vi "FPGA_Amplitude_Pockels_Galvo.vi"(5 "Live(F)/Functional(T)":bool, 6 "Chirp index":i32, 7 "FPGA Type":enum16{"Virtex 5", "Virtex 7"}(ring), 8 "delta_a_dz":dbl[](array[numeric]), 9 "difftime - aodcontrol delay":dbl, 10 "Laser(V) - Vertex 7 Only":dbl[](array[numeric]), 11 "Amplitude":dbl[](array[numeric])) -> (2 "Pockels_Galvo_Params":T1)   [LabVIEW 2020]
uses:
  Controls/Pockels_Galvo_Params.ctl
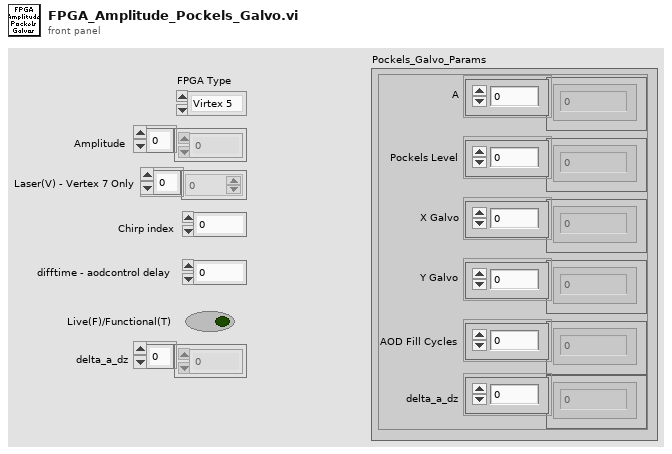
[diagram p1: front panel]
types:
  T1 = typedef "Pockels_Galvo_Params.ctl" = cluster{"A":dbl[], "Pockels Level":dbl[], "X Galvo":dbl[], "Y Galvo":dbl[], "AOD Fill Cycles":dbl[], "delta_a_dz":dbl[]}
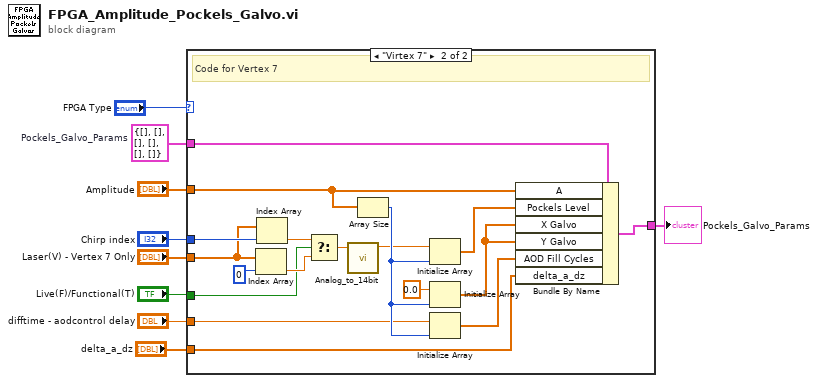
[diagram p0: block diagram]
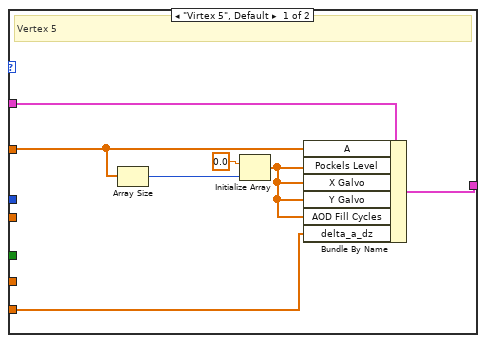
[diagram p2: hidden frame]
diagram:
  w9 = T1 {"A"=[], "Pockels Level"=[], "X Galvo"=[], "Y Galvo"=[], "AOD Fill Cycles"=[], "delta_a_dz"=[]}  # Pockels_Galvo_Params
  n1 = case shown="\"Virtex 7\"" "FPGA Type" {
    tunnel: w9 -> [w15 w25]
    tunnel: "Amplitude" -> [w12 w24]
    tunnel: "Chirp index" -> [_ w23]
    tunnel: "Laser(V) - Vertex 7 Only" -> [_ w22]
    tunnel: "difftime - aodcontrol delay" -> [_ w20]
    tunnel: "Live(F)/Functional(T)" -> [_ w19]
    tunnel: [w16 w18] -> w3
    tunnel: "delta_a_dz" -> [w10 w17]
    frame "Virtex 5", Default {
      # "Vertex 5"
      n2 = Array Size(array=w12) -> (size(s)=w13:i32)
      n3 = Initialize Array(0.0 ("element"), w13) -> (w11:dbl[])
      n4 = Bundle By Name(cluster=w15, "A"=w12, "Pockels Level"=w11, "X Galvo"=w11, "Y Galvo"=w11, "AOD Fill Cycles"=w11, "delta_a_dz"=w10) -> (w16:T1)
    }
    frame "Virtex 7" {
      # "Code for Vertex 7"
      n5 = Index Array(array=w22, index=0) -> (element=w26:dbl)
      n6 = Index Array(array=w22, index=w23) -> (element=w27:dbl)
      n7 = Select(t=w27, s=w19, f=w26) -> (s? t:f=w28:dbl)
      n8 = call "Analog_to_14bit.vi"("Pockels (0-2V)"=w28) -> ("Pockels Level(14 bit)"=w29:dbl)  [unwired: 10 in]
      n9 = Array Size(array=w24) -> (size(s)=w30:i32)
      n10 = Initialize Array(w29, w30) -> (w31:dbl[])
      n11 = Initialize Array(0.0 ("element"), w30) -> (w34:dbl[])
      n12 = Initialize Array(w20, w30) -> (w33:dbl[])
      n13 = Bundle By Name(cluster=w25, "A"=w24, "Pockels Level"=w31, "X Galvo"=w34, "Y Galvo"=w34, "AOD Fill Cycles"=w33, "delta_a_dz"=w17) -> (w18:T1)
    }
  }
  "Pockels_Galvo_Params" <- w3
